vi "DTCControl.Compile.vi"(8 "error in (no error)":errorcluster, 11 "Section Ref in":T4 format="%.0x") -> (0 "error out":errorcluster, 2 "Settings":T1 {"Signal.Cmd.Refs"."Signal Refs" format="%.0x"; "Signal.Cmd.Info"."Signals"."Byte Order" items=["Little Endian", "Big Endian"]; "Signal.Cmd.Info"."Signals"."Data Type" items=["Signed", "Unsigned", "IEEE Float"]; "Settings.Refs"."Signal Refs" format="%.0x"; "Signal.Resp.Refs"."Signal Refs" format="%.0x"; "Signal.Resp.Info"."Signals"."Byte Order" items=["Little Endian", "Big Endian"]; "Signal.Resp.Info"."Signals"."Data Type" items=["Signed", "Unsigned", "IEEE Float"]; "Trigger.Refs"."Signal Refs" format="%.0x"; "Status.Refs"."Signal Refs" format="%.0x"}, 3 "Section Ref out":T4 format="%.0x")   [LabVIEW 2024, in "Diagnostics Addon System Explorer.lvlib"]
uses:
  Diagnostics Addon System Explorer.lvlib
  <vilib>/NI VeriStand/Custom Device API/Custom Device Item Ref.ctl
  Types/Service.Export.ctl
  Types/Frame.Ref.ctl
  Addon Shared/Types/Type.ctl
  Addon Shared/Types/Frame.Compile.ctl
  Addon Shared/Types/Signal.ctl
  Types/FG.Action.ctl
  Signal.FG.vi
  Frame.GetSignalRefs.vi
  Addon Shared/SubVIs/Constants.vi
  <vilib>/NI VeriStand/Custom Device Tools/Custom Device Utility Library/NI VeriStand - Search for Item by GUID.vi
  <vilib>/NI VeriStand/Custom Device API/NI VeriStand - Get Item Children.vi
  <vilib>/NI VeriStand/Custom Device Tools/Custom Device Utility Library/NI VeriStand - Search for Item by Name.vi
  <vilib>/NI/NI VeriStand Advanced SysDef API/SysDef API/SysDef.Property.Set.vi
  <vilib>/NI/NI VeriStand Advanced SysDef API/_SubVIs/SysDef.Property.Set.U32.vi
  <vilib>/NI VeriStand/Custom Device API/NI VeriStand - Get Item Property.vi
  <vilib>/NI VeriStand/Custom Device API/Get Item Property (U32).vi
  <vilib>/NI VeriStand/Custom Device API/NI VeriStand - Get Item Data.vi
  <vilib>/NI/NI VeriStand Advanced SysDef API/_SubVIs/SysDef.Property.Set.DBL.vi
  <vilib>/NI/NI VeriStand Advanced SysDef API/_SubVIs/SysDef.Property.Set.String.vi
  <vilib>/NI VeriStand/Custom Device API/Get Item Property (Double).vi
  <vilib>/NI VeriStand/Custom Device API/Get Item Property (String).vi
  <vilib>/NI VeriStand/Custom Device API/NI VeriStand - Get Custom Device Channel Data.vi
  <vilib>/NI VeriStand/Custom Device Tools/Custom Device Utility Library/Custom Device Utility Library.lvlib
  <vilib>/NI VeriStand/Custom Device API/Custom Device API.lvlib
  Addon Shared/Diagnostics Addon Shared.lvlib
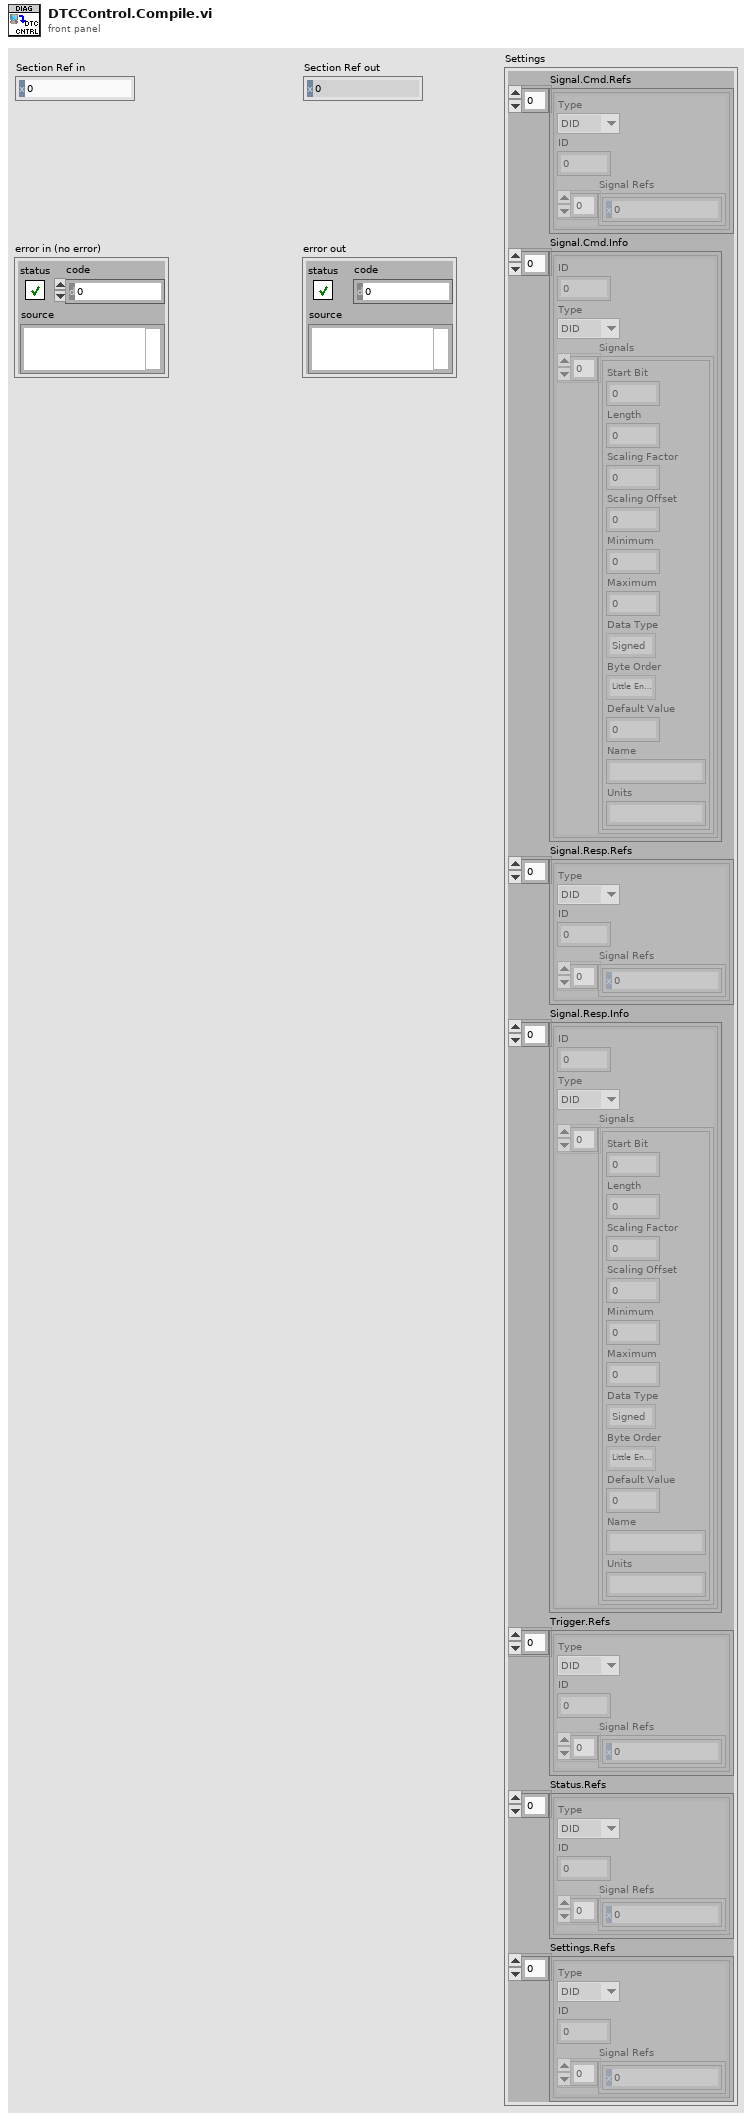
[diagram p1: front panel]
types:
  T1 = typedef "Diagnostics Addon System Explorer.lvlib/Service.Export.ctl" = cluster{"Signal.Cmd.Refs":T2[], "Signal.Cmd.Info":T5[], "Signal.Resp.Refs":T2[], "Signal.Resp.Info":T5[], "Trigger.Refs":T2[], "Status.Refs":T2[], "Settings.Refs":T2[]}
  T2 = typedef "Diagnostics Addon System Explorer.lvlib/Frame.Ref.ctl" = cluster{"Type":T3, "ID":u32, "Signal Refs":T4[]}
  T3 = typedef "Diagnostics Addon Shared.lvlib/Type.ctl" = enum16{"DID", "CDID", "PID", "CPID", "Read Memory", "Write Memory", "IO Control", "Routine Start", "Routine Request", "Routine Stop", "User Defined", "DTC Control", "Clear DTCs", "Read DTCs", "Start DTCs", "DTC Change Count", "Tester Present", "Unlock ECU", "Reset ECU", "Diag Session Control", "Communication Control", "DPID Control", "Poll Control", "Diag Comm Port Control"}
  T4 = typedef "Custom Device API.lvlib/Custom Device Item Ref.ctl" = u64
  T5 = typedef "Diagnostics Addon Shared.lvlib/Frame.Compile.ctl" = cluster{"ID":u32, "Type":T3, "Signals":T6[]}
  T6 = typedef "Diagnostics Addon Shared.lvlib/Signal.ctl" = cluster{"Start Bit":u32, "Length":u32, "Scaling Factor":dbl, "Scaling Offset":dbl, "Minimum":dbl, "Maximum":dbl, "Data Type":u32, "Byte Order":u32, "Default Value":dbl, "Name":string, "Units":string}
  T7 = typedef "Diagnostics Addon System Explorer.lvlib/FG.Action.ctl" = enum16{"Get", "Set"}
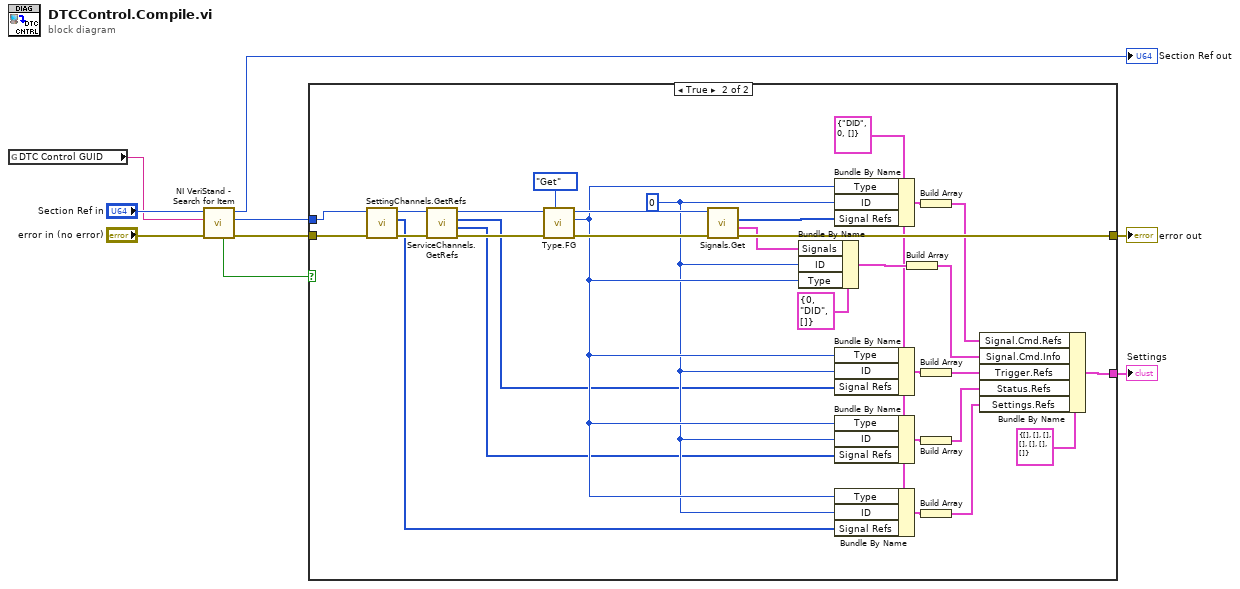
[diagram p0: block diagram]
diagram:
  n1 = global read "Constants.vi" "DTC Control GUID"() -> (w2:string)
  n2 = call-poly <vilib>:"NI VeriStand - Search for Item.vi"("error in"="error in (no error)", "Item GUID"=w2, "Section Ref in"="Section Ref in") -> ("error out"=w4:errorcluster, "Item Ref"=w5:T4, "Section Ref out"=→"Section Ref out":T4, "Found"=w3:bool)  [unwired: 5 in]
  n3 = case shown="True" w3 {
    tunnel: [w10 w41] -> w8
    tunnel: w5 -> [_ w23]
    tunnel: w4 -> [w10 w25]
    tunnel: [_ w29] -> w1
    frame False {
    }
    frame True {
      w18 = 0
      w17 = T2 {"Type"=enum."DID", "ID"=0, "Signal Refs"=[]} ("cluster")
      n4 = call "SettingChannels.GetRefs.vi"("error in (no error)"=w25, "Item Ref in"=w23) -> ("error out"=w28:errorcluster, "Settings"=w14:T4[], "Section Ref out"=w27:T4)  [unwired: 7 in]
      n5 = call "ServiceChannels.GetRefs.vi"("error in (no error)"=w28, "Item Ref in"=w27) -> ("error out"=w26:errorcluster, "Status"=w15:T4[], "Trigger"=w16:T4[], "Section Ref out"=w24:T4)  [unwired: 6 in]
      n6 = call "Type.FG.vi"("Action"=FG.Action."Get", "error in (no error)"=w26, "Device Item Ref in"=w24) -> ("error out"=w34:errorcluster, "Type"=w19:T3, "Device Item Ref out"=w33:T4)  [unwired: 6 in]
      n7 = call "Signals.Get.vi"("error in (no error)"=w34, "Device Item Ref out"=w33) -> ("error out"=w41:errorcluster, "Parameters"=w36:T6[], "Child Refs"=w38:T4[])  [unwired: 6 in, 1 out]
      n8 = Bundle By Name(cluster=T5 {"ID"=0, "Type"=enum."DID", "Signals"=[]} ("PID In"), "Signals"=w36, "ID"=w18, "Type"=w19) -> (w39:T5)
      n9 = Bundle By Name(cluster=w17, "Type"=w19, "ID"=w18, "Signal Refs"=w38) -> (w40:T2)
      n10 = Bundle By Name(cluster=w17, "Type"=w19, "ID"=w18, "Signal Refs"=w16) -> (w22:T2)
      n11 = Bundle By Name(cluster=w17, "Type"=w19, "ID"=w18, "Signal Refs"=w15) -> (w21:T2)
      n12 = Bundle By Name(cluster=w17, "Type"=w19, "ID"=w18, "Signal Refs"=w14) -> (w20:T2)
      n13 = Build Array(w39) -> (w31:T5[])
      n14 = Build Array(w40) -> (w30:T2[])
      n15 = Build Array(w22) -> (w13:T2[])
      n16 = Build Array(w21) -> (w12:T2[])
      n17 = Build Array(w20) -> (w11:T2[])
      n18 = Bundle By Name(cluster=T1 {"Signal.Cmd.Refs"=[], "Signal.Cmd.Info"=[], "Signal.Resp.Refs"=[], "Signal.Resp.Info"=[], "Trigger.Refs"=[], "Status.Refs"=[], "Settings.Refs"=[]}, "Signal.Cmd.Refs"=w30, "Signal.Cmd.Info"=w31, "Trigger.Refs"=w13, "Status.Refs"=w12, "Settings.Refs"=w11) -> (w29:T1)
    }
  }
  "error out" <- w8
  "Settings" <- w1
